vi "Configure Channel Summation.vi"(6 "Channel Ratio (0.5)":dbl=0.5, 7 "Enable Channel Summation (T: Enable)":bool=TRUE, 8 "error in (no error)":errorcluster, 9 "External Sum Input Attenuation (0: 0 dBm)":u16(ring) items=["0 dBm", "10 dBm", "20 dBm", "30 dBm", "40 dBm", "50 dBm"], 10 "Channel Summation Source (0: External Sum)":u16(ring) items=["External Sum", "Previous Channel"], 11 "VISA resource name":refnum<visa-resource-name>) -> (0 "error out":errorcluster, 3 "VISA resource name out":refnum<visa-resource-name>)   [LabVIEW 2015, in "Fluke 28x Series.lvlib"]
doc: "Configures the instrument for outputting a waveform comprising the sum of any two channels. \n\n External Sum cannot be used with Internal Modulation and Internal Sum cannot be used with Internal Modulation. If these conditions do occur, a \"Sum or modulation conflict\" error will be output. \n\n<b>Note</b>: This VI applies only to multichannel instruments, i.e. Fluke 282 and Fluke 284."
uses:
  <instrlib>/Fluke 28x Series/Fluke 28x Series.lvlib
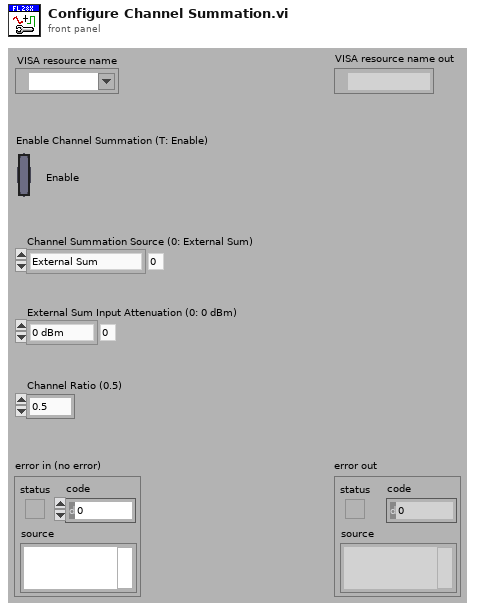
[diagram p1: front panel]
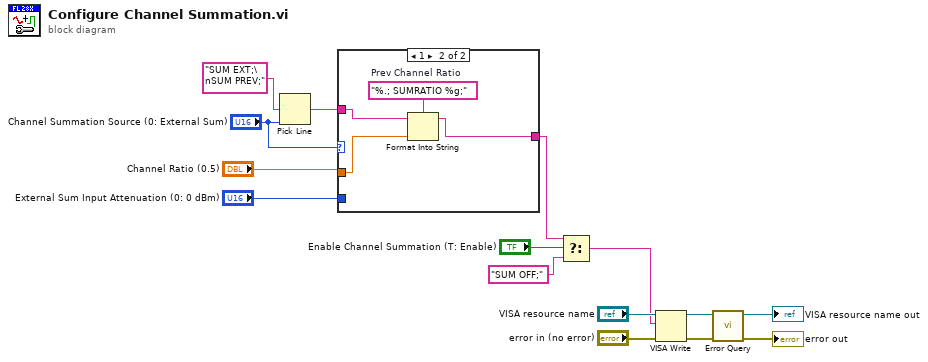
[diagram p0: block diagram]
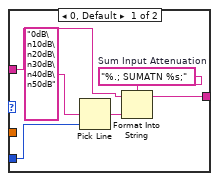
[diagram p2: hidden frame]
diagram:
  n1 = Pick Line(multi-line string="SUM EXT;\nSUM PREV;", line index="Channel Summation Source (0: External Sum)") -> (output string=w6:string)  [unwired: 1 in]
  n2 = case shown="1" "Channel Summation Source (0: External Sum)" {
    tunnel: [w18 w24] -> w4
    tunnel: w6 -> [w17 w23]
    tunnel: "Channel Ratio (0.5)" -> [_ w22]
    tunnel: "External Sum Input Attenuation (0: 0 dBm)" -> [w16 _]
    frame 0, Default {
      w19 = "%.; SUMATN %s;"  # Sum Input Attenuation
      n3 = Pick Line(multi-line string="0dB\n10dB\n20dB\n30dB\n40dB\n50dB", line index=w16) -> (output string=w20:string)  [unwired: 1 in]
      n4 = Format Into String(format string=w19, initial string=w17, w20) -> (resulting string=w18:string)  [unwired: 1 in, 1 out]
    }
    frame 1 {
      w25 = "%.; SUMRATIO %g;"  # Prev Channel Ratio
      n5 = Format Into String(format string=w25, initial string=w23, w22) -> (resulting string=w24:string)  [unwired: 1 in, 1 out]
    }
  }
  n6 = Select(t=w4, s="Enable Channel Summation (T: Enable)", f="SUM OFF;") -> (s? t:f=w1:string)
  n7 = VISA Write(VISA resource name="VISA resource name", write buffer=w1, error in (no error)="error in (no error)") -> (VISA resource name out=w14:refnum<visa-resource-name>, error out=w13:errorcluster)  [unwired: 1 out]
  n8 = call <instrlib>:"Error Query.vi"("error in (no error)"=w13, "VISA resource name"=w14) -> ("error out"=→"error out":errorcluster, "VISA resource name out"=→"VISA resource name out":refnum<visa-resource-name>)  [unwired: 6 in, 2 out]
